vi "Inverted Rotation.vi"(8 "error in (no error)":errorcluster, 10 "Rotation in":dbl, 11 "FlexWorktable in":refnum<class "FlexWorktable.lvclass">) -> (0 "error out":errorcluster, 2 "Rotation out":dbl, 3 "FlexWorktable out":refnum<class "FlexWorktable.lvclass">)   [LabVIEW 2017, in "FlexWorktable.lvclass"]
uses:
  FlexWorktable.lvclass
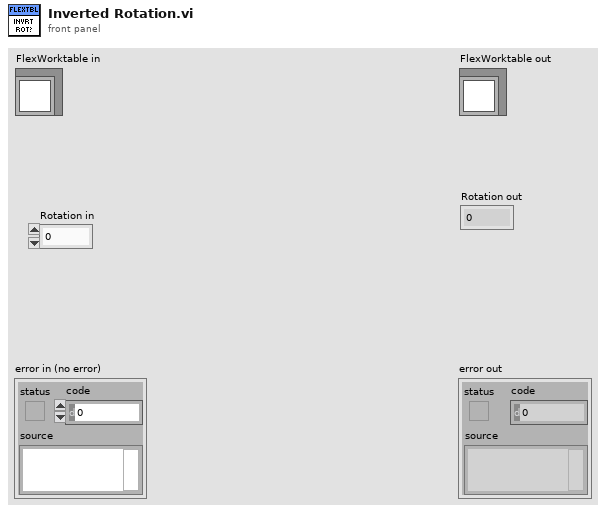
[diagram p1: front panel]
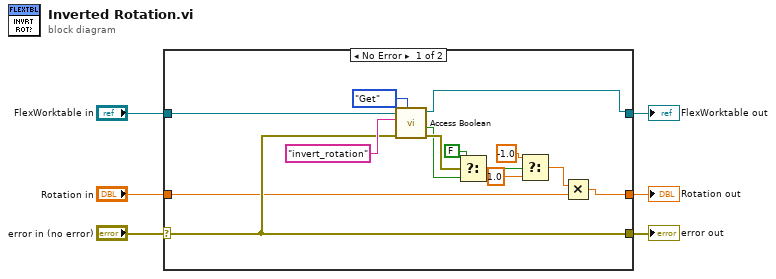
[diagram p0: block diagram]
diagram:
  n1 = case shown="No Error" "error in (no error)" {
    selector: "error in (no error)" -> [w11 w23]
    tunnel: [w11 w23] -> w5
    tunnel: [w7 w22] -> w3
    tunnel: "FlexWorktable in" -> [w13 w22]
    tunnel: "Rotation in" -> [w10 w21]
    tunnel: [w8 w21] -> w1
    frame No Error {
      n2 = call-dynamic "Access Boolean.vi"("Get/Set"=enum16{"Get", "Set"}."Get", "error in (no error)"=w11, "Key"="invert_rotation", "FlexWorktable in"=w13) -> ("error out"=w18:errorcluster, "Value out"=w17:bool, "FlexWorktable out"=w7:refnum<class "FlexWorktable.lvclass">)  [unwired: 5 in]
      n3 = Select(t=FALSE, s=w18, f=w17) -> (s? t:f=w15:bool)
      n4 = Select(t=-1.0, s=w15, f=1.0) -> (s? t:f=w9:dbl)
      n5 = Multiply(x=w9, y=w10) -> (x*y=w8:dbl)
    }
    frame Error {
    }
  }
  "error out" <- w5
  "FlexWorktable out" <- w3
  "Rotation out" <- w1
